vi "ms Delay.vi"(1 "miliseconds to wait":u32, 2 "error in (no error)":errorcluster) -> (5 "millisecond timer value":u32, 7 "error out":errorcluster)   [LabVIEW 2025, in "Chroma 19052.lvlib"]
uses:
  <instrlib>/Chroma 19052/Chroma 19052.lvlib
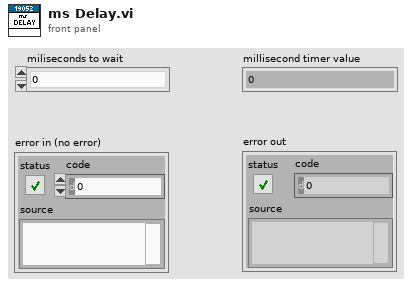
[diagram p1: front panel]
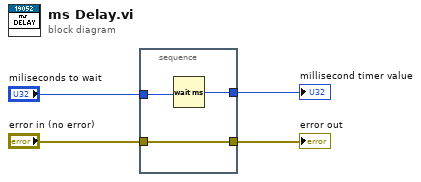
[diagram p0: block diagram]
diagram:
  n1 = stacked-sequence {
    tunnel: "miliseconds to wait" -> [w7]
    tunnel: "error in (no error)" -> [w6]
    tunnel: [w6] -> w1
    tunnel: [w5] -> w3
    frame #0 {
      n2 = Wait (ms)(milliseconds to wait=w7) -> (millisecond timer value=w5:u32)
    }
  }
  "millisecond timer value" <- w3
  "error out" <- w1
